vi "SeqNum Analysis.vi"(5 "SeqNum_In":u16, 6 "Buffer_In":u8[](array[numeric])) -> (0 "Status":u8, 1 "RF Quality":dbl format="%#_4g", 2 "SeqNum_Out":u8, 3 "Buffer_Out":u8[](array[numeric]), 4 "Packet Lost":bool)   [LabVIEW 2013]
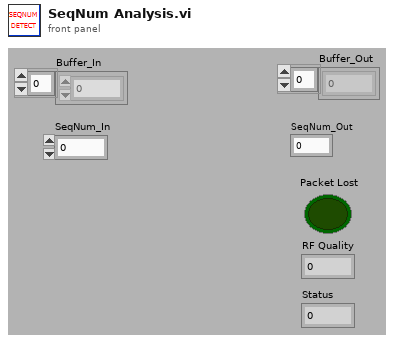
[diagram p1: front panel]
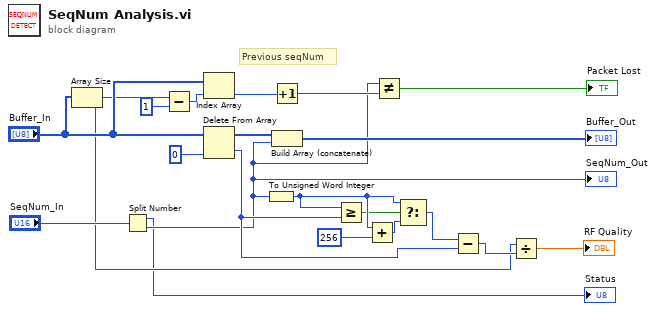
[diagram p0: block diagram]
diagram:
  # "Previous seqNum"
  n1 = Array Size(array="Buffer_In") -> (size(s)=w2:i32)
  n2 = Split Number(x="SeqNum_In") -> (hi(x)=→"Status":u8, lo(x)=w3:u8)
  "SeqNum_Out" <- w3
  n3 = Subtract(x=w2, y=1) -> (x-y=w5:i32)
  n4 = Index Array(array="Buffer_In", index=w5) -> (element=w4:u8)
  n5 = Delete From Array(array="Buffer_In", index=0) -> (deleted portion=w14:u8, array with subset deleted=w11:u8[])  [unwired: 1 in]
  n6 = To Unsigned Word Integer(number=w3) -> (unsigned 16bit integer=w16:u16)
  n7 = Increment(x=w4) -> (x+1=w9:u8)
  n8 = Build Array (concatenate)(w11, w3) -> (→"Buffer_Out":u8[])
  n9 = Greater Or Equal?(x=w16, y=w14) -> (x >= y?=w15:bool)
  n10 = Add(x=w16, y=u16 256) -> (x+y=w18:u16)
  n11 = Not Equal?(x=w3, y=w9) -> (x != y?=→"Packet Lost":bool)
  n12 = Select(t=w16, s=w15, f=w18) -> (s? t:f=w19:u16)
  n13 = Subtract(x=w19, y=w14) -> (x-y=w21:u16)
  n14 = Divide(x=w2, y=w21) -> (x/y=→"RF Quality":dbl)
